vi "Scale Raw Data_Array.vi"(7 "Wfm Data":waveform(sgl)[](array[waveform])) -> (8 "Wfm Data out":waveform(sgl)[](array[waveform]))   [LabVIEW 2014]
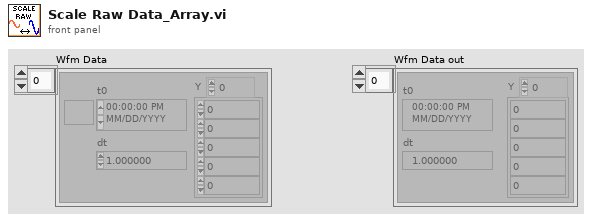
[diagram p1: front panel]
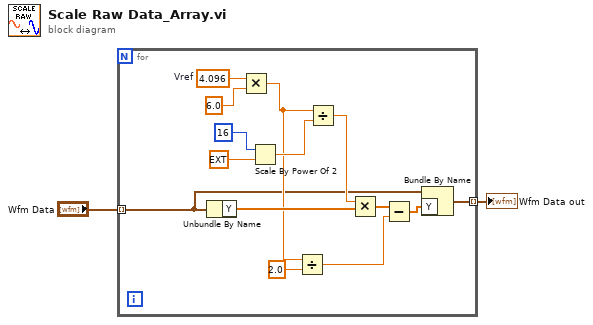
[diagram p0: block diagram]
diagram:
  n1 = for {
    tunnel: "Wfm Data" -> [w4] mode=indexing
    tunnel: [w3] -> w1 mode=indexing
    w14 = 4.096  # Vref
    n2 = Unbundle By Name(w4) -> ("Y"=w10:sgl[])
    n3 = Multiply(x=w14, y=6.0) -> (x*y=w8:dbl)
    n4 = Scale By Power Of 2(n=i16 16, x=ext 1.0) -> (x*2^n=w12:ext)
    n5 = Divide(x=w8, y=2.0) -> (x/y=w6:dbl)
    n6 = Divide(x=w8, y=w12) -> (x/y=w11:ext)
    n7 = Multiply(x=w11, y=w10) -> (x*y=w9:ext[])
    n8 = Subtract(x=w9, y=w6) -> (x-y=w5:ext[])
    n9 = Bundle By Name(cluster=w4, "Y"=w5) -> (w3:waveform(sgl))
  }
  "Wfm Data out" <- w1
